vi "Load Settings from Report.vi"() -> ()   [LabVIEW 2014, in "POLARIS IMAQ Display.xctl"]
uses:
  POLARIS IMAQ Display.xctl
panel:
  in  "ref":refnum<vi>
  in  "Select Report File":path
  in  "Stop":bool
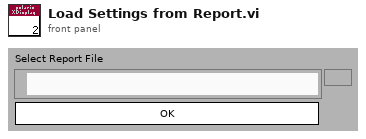
[diagram p1: front panel]
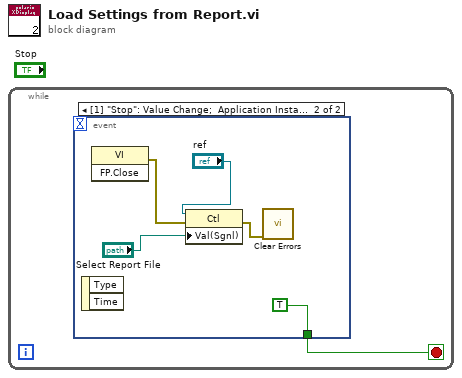
[diagram p0: block diagram]
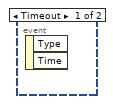
[diagram p2: hidden frame]
diagram:
  n1 = while {
    stop <- w1 stop-if-true
    n2 = event shown="[1] \"Stop\": Value Change;  Application Instance Close" {
      selector: _ -> [_ _]
      dyn-events: _ -> [_ _]
      timeout: _ -> [_ _]
      tunnel: [_ TRUE] -> w1
      event Timeout {
        n3 = event-data() -> ()  [unwired: 1 in, 2 out]
      }
      event "Stop": Value Change; Application Instance Close {
        n4 = event-data() -> ()  [unwired: 1 in, 2 out]
        n5 = invoke class="VI" method="FP.Close"() -> (error out=w3:errorcluster)  [unwired: 3 in, 2 out]
        n6 = property class="Ctl"(reference="ref", error in=w3, "Val(Sgnl)"="Select Report File") -> (error out=w4:errorcluster)  [unwired: 1 out]
        n7 = call <vilib>:"Clear Errors.vi"("error in (no error)"=w4) -> ()  [unwired: 5 in, 2 out]
      }
    }
  }
